vi "API - Create Rx Section.vi"(8 "error in (no error)":errorcluster, 10 "Packet Info":T1[](array[typedef]) {"Channels"."Destination Ref" format="%.0x"}, 11 "Rx Section Ref In":T3 format="%.0x") -> (0 "error out":errorcluster, 3 "Rx Section Ref Out":T3 format="%.0x")   [LabVIEW 2016, in "UDP-Custom-Device System Explorer.lvlib"]
uses:
  UDP-Custom-Device System Explorer.lvlib
  <vilib>/NI Veristand/Custom Device API/Custom Device Item Ref.ctl
  Types/TypeDef - Rx Packet Data.ctl
  TypeDef - Channel Data.ctl
  Shared/DataTypes.ctl
  <vilib>/NI VeriStand/Custom Device API/Custom Device API.lvlib
  Shared/UDP-Custom-Device Shared.lvlib
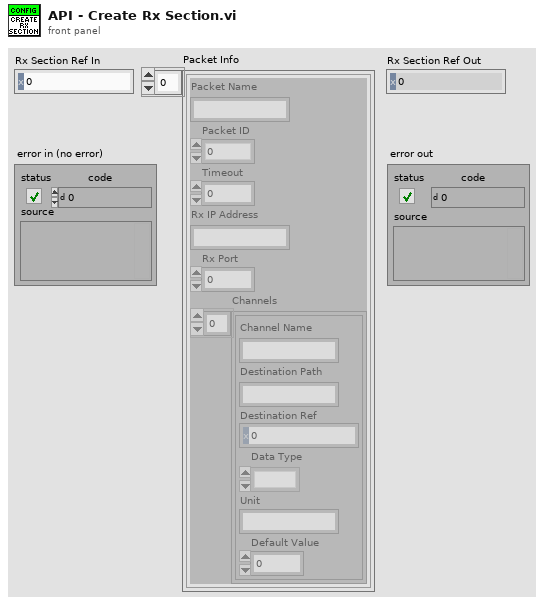
[diagram p1: front panel]
types:
  T1 = typedef "UDP-Custom-Device System Explorer.lvlib/TypeDef - Rx Packet Data.ctl" = cluster{"Packet Name":string, "Packet ID":i32, "Timeout":i32, "Rx IP Address":string, "Rx Port":i32, "Channels":T2[]}
  T2 = typedef "UDP-Custom-Device System Explorer.lvlib/TypeDef - Channel Data.ctl" = cluster{"Channel Name":string, "Destination Path":string, "Destination Ref":T3, "Data Type":T4, "Unit":string, "Default Value":dbl}
  T3 = typedef "Custom Device API.lvlib/Custom Device Item Ref.ctl" = u64
  T4 = typedef "UDP-Custom-Device Shared.lvlib/DataTypes.ctl" = enum16{""}
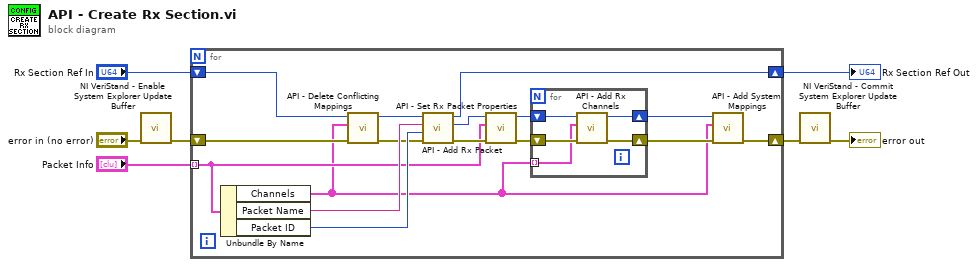
[diagram p0: block diagram]
diagram:
  n1 = call <vilib>:"NI VeriStand - Enable System Explorer Update Buffer.vi"("error in (no error)"="error in (no error)") -> ("error out"=w3:errorcluster)  [unwired: 10 in]
  n2 = for {
    tunnel: "Packet Info" -> [w15] mode=indexing
    shift-right: [w11] -> w2
    shift-left: w3 -> [w18]
    shift-right: [w9] -> w5
    shift-left: "Rx Section Ref In" -> [w21]
    n3 = Unbundle By Name(w15) -> ("Channels"=w8:T2[], "Packet Name"=w23:string, "Packet ID"=w22:i32)
    n4 = call "API - Delete Conflicting Mappings.vi"("error in (no error)"=w18, "Channels"=w8, "Rx Section Ref In"=w21) -> ("error out"=w19:errorcluster, "Rx Section Ref Out"=w20:T3)  [unwired: 7 in]
    n5 = call "API - Add Rx Packet.vi"("error in (no error)"=w19, "New Packet ID"=w22, "New Packet Name"=w23, "Item Ref in"=w20) -> ("error out"=w17:errorcluster, "New Packet Ref"=w16:T3, "Item Ref Out"=w9:T3)  [unwired: 5 in]
    n6 = call "API - Set Rx Packet Properties.vi"("error in (no error)"=w17, "Rx Packet Info"=w15, "Packet Ref In"=w16) -> ("error out"=w14:errorcluster, "Packet Ref Out"=w13:T3)  [unwired: 7 in]
    n7 = for {
      shift-right: [w25] -> w12
      shift-left: w14 -> [w27]
      shift-right: [w24] -> w10
      shift-left: w13 -> [w28]
      tunnel: w8 -> [w26] mode=indexing
      n8 = call "API - Add Rx Channels.vi"("error in (no error)"=w27, "Channel Data"=w26, "Packet Ref In"=w28) -> ("error out"=w25:errorcluster, "Packet Ref Out"=w24:T3)  [unwired: 6 in, 1 out]
    }
    n9 = call "API - Add System Mappings.vi"("error in (no error)"=w12, "Channels"=w8, "Rx Section Ref In"=w10) -> ("error out"=w11:errorcluster)  [unwired: 7 in, 1 out]
  }
  "Rx Section Ref Out" <- w5
  n10 = call <vilib>:"NI VeriStand - Commit System Explorer Update Buffer.vi"("error in (no error)"=w2) -> ("error out"=→"error out":errorcluster)  [unwired: 10 in]
